vi "Pickering 40-295 Initialization.vi"(8 "error in (no error)":errorcluster, 10 "Custom XML":string, 11 "Device Item Ref in":T1 format="%.0x") -> (0 "error out":errorcluster, 3 "Device Item Ref out":T1 format="%.0x")   [LabVIEW 2014, in "Pickering 40-295.lvlib"]
doc: "The Initialization VI is used to populate the tree with the most important elements. It is mandatory to add at least the main page!\nBy calling the Add Items VI make sure that sections are added before the channels. Also make sure that for nested sections each individual section is created (from top to bottwom)."
uses:
  Pickering 40-295.lvlib
  <vilib>/NI Veristand/Custom Device API/Custom Device Item Ref.ctl
  <vilib>/NI Veristand/Custom Device API/Custom Device Loop Type.ctl
  <vilib>/NI Veristand/Custom Device API/Custom Device Channel Type.ctl
  <vilib>/NI Veristand/Custom Device API/Custom Device Channel.ctl
  <vilib>/NI Veristand/Custom Device API/Set Item Property (String).vi
  <vilib>/NI Veristand/Custom Device API/Custom Device API.lvlib
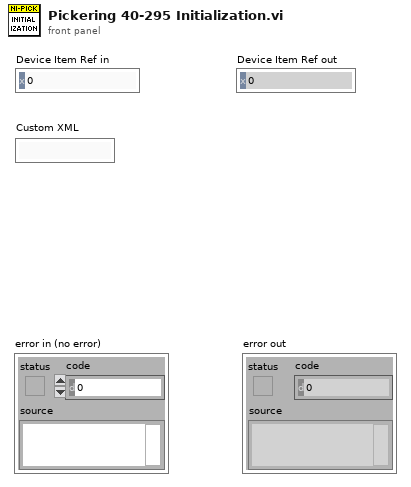
[diagram p1: front panel]
types:
  T1 = typedef "Custom Device API.lvlib/Custom Device Item Ref.ctl" = u64
  T2 = typedef "Custom Device API.lvlib/Custom Device Channel.ctl" = cluster{"Type":T3, "Units":string, "Default Value":dbl, "Faultable":bool, "Scalable":bool}
  T3 = typedef "Custom Device API.lvlib/Custom Device Channel Type.ctl" = enum16{"Input", "Output"}
  T4 = typedef "Custom Device API.lvlib/Custom Device Loop Type.ctl" = enum32{"While Loop", "Timed Loop"}
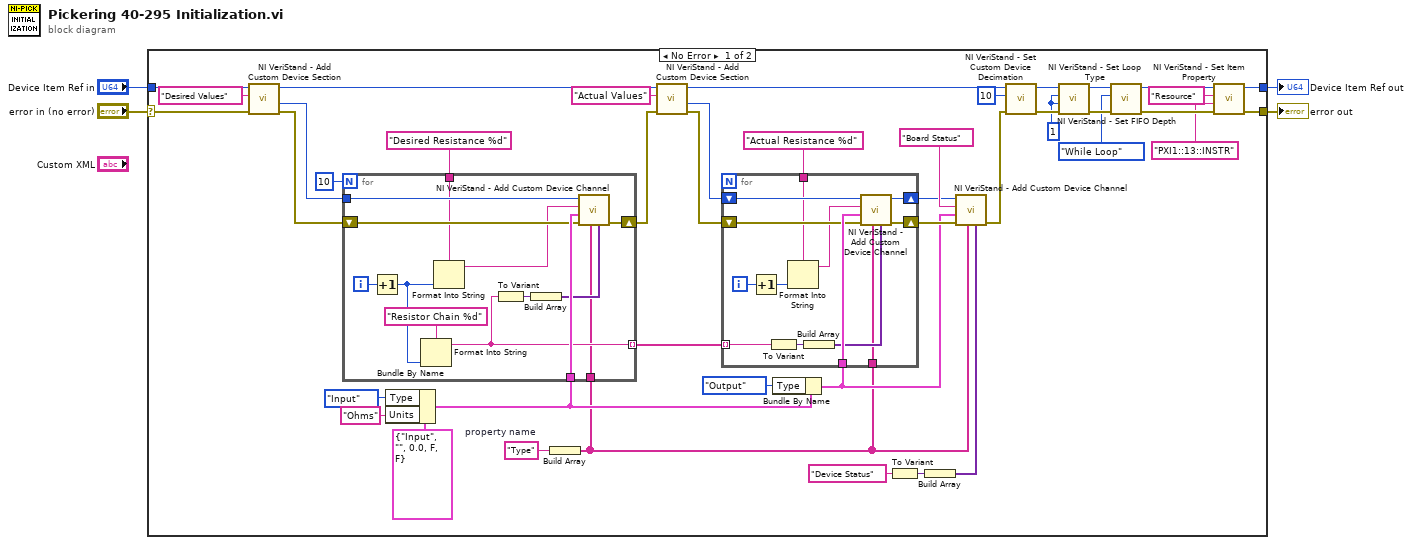
[diagram p0: block diagram]
diagram:
  n1 = case shown="No Error" "error in (no error)" {
    selector: "error in (no error)" -> [w21 w74]
    tunnel: [w10 w74] -> w4
    tunnel: [w11 w75] -> w3
    tunnel: "Device Item Ref in" -> [w40 w75]
    frame No Error {
      w38 = "Type"  # property name
      w44 = u32 1 ("Size FIFO Read (10)")
      n2 = call <vilib>:"NI VeriStand - Add Custom Device Section.vi"("error in (no error)"=w21, "Section Name"="Desired Values", "Parent Ref in"=w40) -> ("error out"=w33:errorcluster, "Section Ptr"=w37:T1, "Parent Ref out"=w31:T1)  [unwired: 4 in, 2 out]
      n3 = Bundle By Name(cluster=T2 {"Type"=enum."Input", "Units"="", "Default Value"=0.0, "Faultable"=FALSE, "Scalable"=FALSE} ("Channel"), "Type"=Custom_Device_Channel_Type."Input", "Units"="Ohms") -> (w26:T2)
      n4 = Build Array(w38) -> (w7:string[])
      n5 = for {
        N: 10 -> [_]
        tunnel: w37 -> [w70]
        tunnel: w7 -> [w61]
        tunnel: "Desired Resistance %d" ("String") -> [w68]
        tunnel: w26 -> [w73]
        shift-right: [w66] -> w30
        shift-left: w33 -> [w71]
        tunnel: [w62] -> w6 mode=indexing
        i -> [w69]
        n6 = Increment(x=w69) -> (x+1=w63:i32)
        n7 = Format Into String(format string="Resistor Chain %d" ("String"), w63) -> (resulting string=w62:string)  [unwired: 2 in, 1 out]
        n8 = Format Into String(format string=w68, w63) -> (resulting string=w67:string)  [unwired: 2 in, 1 out]
        n9 = To Variant(anything=w62) -> (Variant=w64:variant)
        n10 = Build Array(w64) -> (w72:variant[])
        n11 = call <vilib>:"NI VeriStand - Add Custom Device Channel.vi"("Property Values"=w72, "Property names"=w61, "error in (no error)"=w71, "Channel"=w73, "Channel Name"=w67, "Parent Ref in"=w70) -> ("error out"=w66:errorcluster)  [unwired: 2 in, 3 out]
      }
      n12 = call <vilib>:"NI VeriStand - Add Custom Device Section.vi"("error in (no error)"=w30, "Section Name"="Actual Values", "Parent Ref in"=w31) -> ("error out"=w16:errorcluster, "Section Ptr"=w19:T1, "Parent Ref out"=w23:T1)  [unwired: 4 in, 2 out]
      n13 = Bundle By Name(cluster=w26, "Type"=Custom_Device_Channel_Type."Output") -> (w15:T2)
      n14 = for {
        tunnel: w7 -> [w56]
        tunnel: "Actual Resistance %d" ("String") -> [w54]
        tunnel: w15 -> [w60]
        shift-right: [w52] -> w17
        shift-left: w16 -> [w58]
        shift-right: [w49] -> w18
        shift-left: w19 -> [w57]
        tunnel: w6 -> [w48] mode=indexing
        i -> [w55]
        n15 = Increment(x=w55) -> (x+1=w50:i32)
        n16 = To Variant(anything=w48) -> (Variant=w51:variant)
        n17 = Format Into String(format string=w54, w50) -> (resulting string=w53:string)  [unwired: 2 in, 1 out]
        n18 = Build Array(w51) -> (w59:variant[])
        n19 = call <vilib>:"NI VeriStand - Add Custom Device Channel.vi"("Property Values"=w59, "Property names"=w56, "error in (no error)"=w58, "Channel"=w60, "Channel Name"=w53, "Parent Ref in"=w57) -> ("error out"=w52:errorcluster, "Parent Ref out"=w49:T1)  [unwired: 2 in, 2 out]
      }
      n20 = To Variant(anything="Device Status" ("String")) -> (Variant=w29:variant)
      n21 = Build Array(w29) -> (w24:variant[])
      n22 = call <vilib>:"NI VeriStand - Add Custom Device Channel.vi"("Property Values"=w24, "Property names"=w7, "error in (no error)"=w17, "Channel"=w15, "Channel Name"="Board Status" ("String"), "Parent Ref in"=w18) -> ("error out"=w22:errorcluster)  [unwired: 2 in, 3 out]
      n23 = call <vilib>:"NI VeriStand - Set Custom Device Decimation.vi"("error in (no error)"=w22, "Decimation"=10, "Device Ref in"=w23) -> ("error out"=w45:errorcluster, "Device Ref out"=w46:T1)  [unwired: 7 out]
      n24 = call <vilib>:"NI VeriStand - Set FIFO Depth.vi"("error in (no error)"=w45, "Size FIFO Sink (1)"=w44, "Size FIFO Source (1)"=w44, "Device Ref in"=w46) -> ("error out"=w43:errorcluster, "Device Ref out"=w42:T1)  [unwired: 6 out]
      n25 = call <vilib>:"NI VeriStand - Set Loop Type.vi"("error in (no error)"=w43, "Loop type"=Custom_Device_Loop_Type."While Loop", "Device Ref in"=w42) -> ("error out"=w12:errorcluster, "Device Ref out"=w13:T1)  [unwired: 1 in, 6 out]
      n26 = call-poly <vilib>:"NI VeriStand - Set Item Property.vi"("error in (no error)"=w12, "Value"="PXI1::13::INSTR" ("Section Name"), "Property Name"="Resource" ("Section Name"), "Item Ref in"=w13) -> ("error out"=w10:errorcluster, "Item Ref out"=w11:T1)  [unwired: 6 out]
    }
    frame Error {
    }
  }
  "error out" <- w4
  "Device Item Ref out" <- w3
